vi "ws Auth Get.vi"(8 "error in (no error)":errorcluster) -> (0 "error out":errorcluster, 3 "Authorization":T1)   [LabVIEW 2011]
uses:
  license/Authorization Data.ctl
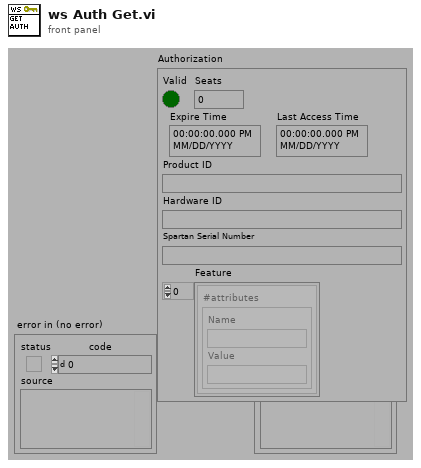
[diagram p1: front panel]
types:
  T1 = typedef "Authorization Data.ctl" = cluster{"Valid":bool, "Seats":i32, "Expire Time":timestamp, "Last Access Time":timestamp, "Product ID":string, "Hardware ID":string, "Spartan Serial Number":string, "Feature":cluster{"#attributes":cluster{"Name":string, "Value":string}}[]}
  T2 = typedef "Authorization Data.ctl" = cluster{"Seats":i32, "Authorizations":bool[], "Site Code":string}
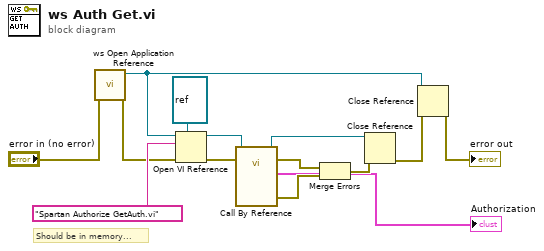
[diagram p0: block diagram]
diagram:
  # "Should be in memory..."
  n1 = call "ws Open Application Reference.vi"("error in (no error)"="error in (no error)") -> ("error out"=w2:errorcluster, "application reference"=w1:refnum<vi>)  [unwired: 9 in]
  n2 = Open VI Reference(type specifier VI Refnum (for type only)=refnum<vi> refnum, application reference (local)=w1, vi path="Spartan Authorize GetAuth.vi", error in (no error)=w2) -> (vi reference=w11:refnum<vi>, error out=w12:errorcluster)  [unwired: 2 in]
  n3 = call-by-ref "?"(reference=w11, error in=w12) -> (reference out=w10:refnum<vi>, error out=w9:errorcluster, 0:"error out"=w6:errorcluster, "Authorization"=→"Authorization":T2)  [unwired: 6 in]
  n4 = Merge Errors(w9, w6) -> (w8:errorcluster)
  n5 = Close Reference(reference=w10, error in (no error)=w8) -> (error out=w14:errorcluster)
  n6 = Close Reference(reference=w1, error in (no error)=w14) -> (error out=→"error out":errorcluster)
